vi "Create Engine Folder and Copy RT Template.vi"(8 "error in (no error)":errorcluster, 9 "Project Root":path, 10 "Project Name":string, 11 "CD Template":refnum<class "NIVS_PPL_Inline HW Interface.lvclass">) -> (0 "error out":errorcluster)   [LabVIEW 2019, in "NIVS_PPL_Inline HW Interface.lvclass"]
uses:
  NIVS_PPL_Inline HW Interface.lvclass
  NIVS_Consolidated_CDW_MetaDataObj/CD Engine lvlib.ctl
  NIVS_Consolidated_CDW_MetaDataObj/Common.ctl
  NIVS_Consolidated_CDW_MetaDataObj/CD Engine lvlib.vi
  NIVS_Consolidated_CDW_MetaDataObj/Common.vi
  NIVS_Consolidated_CDW_MetaDataObj/NIVS_Consolidated_CDW_MetaDataObj.lvclass
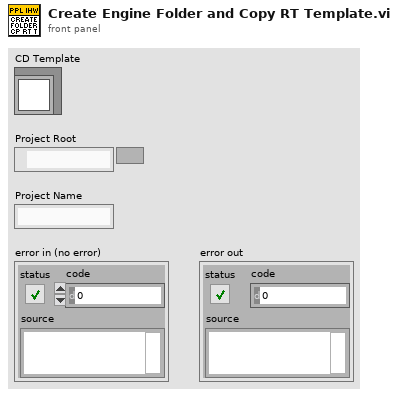
[diagram p1: front panel]
types:
  T1 = typedef "NIVS_Consolidated_CDW_MetaDataObj.lvclass/CD Engine lvlib.ctl" = enum16{"LibraryFileName", "LibraryFolderName", "Engine.FolderName", "Engine.Init.FolderName", "Engine.Run.FolderName", "Engine.Shutdown.FolderName", "Types.FolderName", "Engine.RT Driver VI.TemplatePath", "Engine.RT Driver VI.FileName", "Engine.PPL.RT Driver VI_InlineAsync.FileName", "Engine.RTStateVariables.Name", "Engine.PPL.RTStateVariables.Name", "Engine.RTStateVariables.Name.NoExtension", "Engine.Async.NameExtension", "Engine.Async.TemplateName", "Engine.PPL.Async.TemplateName", "Engine.PPL.Async.InitVSGlobals.Name", "Engine.PPL.RT Driver VI_Inline.FileName"}
  T2 = typedef "NIVS_Consolidated_CDW_MetaDataObj.lvclass/Common.ctl" = enum16{"ProjectName", "TemplatesFolderName", "PPLTemplatesFolderName", "ProjectTemplatePathAndName", "ProjectPPLTemplatePathAndName", "TimingAndSyncFolderName", "CustomDeviceFolderName", "PathToTemplates", "PathToPPLTemplates", "PathToExplorerPPLTemplates", "PathToEnginePPLTemplates", "PathToConfigurationFile", "ProjectConfigurationName"}
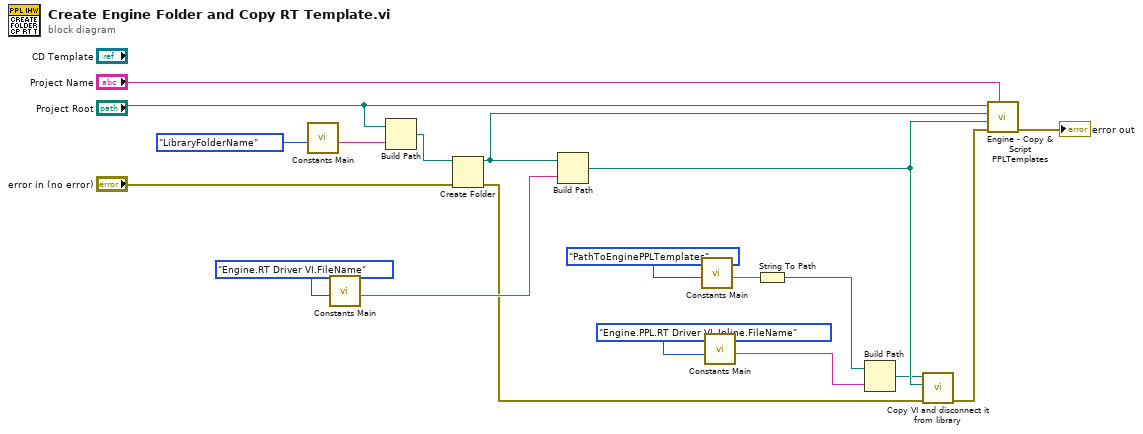
[diagram p0: block diagram]
diagram:
  n1 = call-poly "Constants Main.vi"("Action"=CD_Engine_lvlib."LibraryFolderName") -> ("Output"=w11:string)  [unwired: 10 in]
  n2 = call-poly "Constants Main.vi"("Action"=CD_Engine_lvlib."Engine.RT Driver VI.FileName") -> ("Output"=w7:string)  [unwired: 10 in]
  n3 = Build Path(base path="Project Root", name or relative path=w11) -> (appended path=w13:path)
  n4 = Create Folder(path (use dialog)=w13, error in="error in (no error)") -> (created path=w15:path, error out=w5:errorcluster)  [unwired: 1 in, 1 out]
  n5 = Build Path(base path=w15, name or relative path=w7) -> (appended path=w16:path)
  n6 = call-poly "Constants Main.vi"("Action"=Common."PathToEnginePPLTemplates") -> ("Output"=w8:string)  [unwired: 10 in]
  n7 = call-poly "Constants Main.vi"("Action"=CD_Engine_lvlib."Engine.PPL.RT Driver VI_Inline.FileName") -> ("Output"=w18:string)  [unwired: 10 in]
  n8 = String To Path(string=w8) -> (path=w14:path)
  n9 = Build Path(base path=w14, name or relative path=w18) -> (appended path=w9:path)
  n10 = call "Copy VI and disconnect it from library.vi"("error in (no error)"=w5, "VI Target Path"=w16, "VI Source Path"=w9) -> ("error out"=w17:errorcluster)  [unwired: 8 in]
  n11 = call "Engine - Copy & Script PPLTemplates.vi"("CD Name"="Project Name", "error in (no error)"=w17, "RT Driver VI Path"=w16, "RT Driver Folder Path"=w15, "CD Source Folder Path"="Project Root") -> ("error out"=→"error out":errorcluster)  [unwired: 6 in]
